vi "ClientRefnum.vi"(3 "error in (no error)":errorcluster) -> (16 "OPC UA client refnum out":refnum<k21>, 17 "error out":errorcluster)   [LabVIEW 2014, in "OCPUA Client(UtilityMode)(dev).lvlib"]
uses:
  OCPUA Client(UtilityMode)(dev).lvlib
  _op(client).ctl
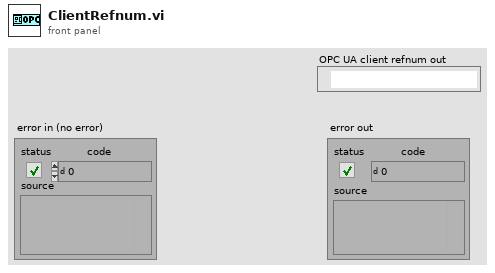
[diagram p1: front panel]
types:
  T1 = typedef "OCPUA Client(UtilityMode)(dev).lvlib/_op(client).ctl" = enum16{"Connect Server", "Get Client Refnum", "Disconnect Server"}
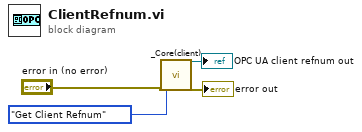
[diagram p0: block diagram]
diagram:
  n1 = call "_Core(client).vi"("error in (no error)"="error in (no error)", "Op"=_op(client)."Get Client Refnum") -> ("OPC UA client refnum out"=→"OPC UA client refnum out":refnum<k21>, "error out"=→"error out":errorcluster)  [unwired: 21 in, 3 out]
